vi "dfd_Get Filter Factor And Type From LM.vi"(8 "M":i32, 11 "L":i32) -> (0 "Factor":string, 3 "Type":string)   [LabVIEW 2017, in "NI_DigFilterLicensed.lvlib"]
uses:
  <vilib>/addons/Digital Filter Design/NI_DigFilterLicensed.lvlib
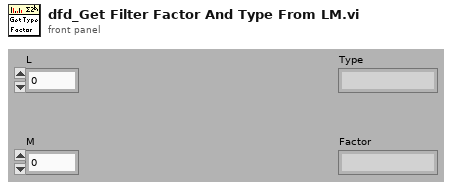
[diagram p1: front panel]
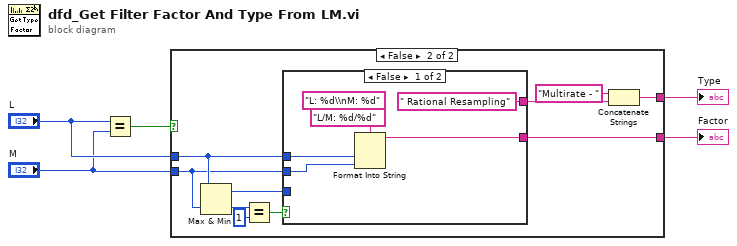
[diagram p0: block diagram]
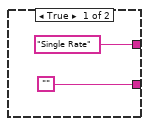
[diagram p2: hidden frame]
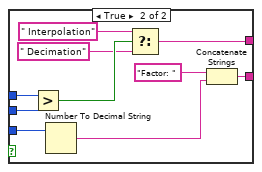
[diagram p3: hidden frame]
diagram:
  n1 = Equal?(x="L", y="M") -> (x = y?=w5:bool)
  n2 = case shown="False" w5 {
    tunnel: "L" -> [_ w13]
    tunnel: "M" -> [_ w12]
    tunnel: ["" w8] -> w1
    tunnel: ["Single Rate" w9] -> w2
    frame True {
    }
    frame False {
      n3 = Max & Min(x=w13, y=w12) -> (max(x,y)=w14:i32, min(x,y)=w16:i32)
      n4 = Equal?(x=w16, y=1) -> (x = y?=w17:bool)
      n5 = case shown="False" w17 {
        tunnel: w14 -> [_ w32]
        tunnel: [w20 w30] -> w8
        tunnel: w13 -> [w22 w28]
        tunnel: w12 -> [w21 w29]
        tunnel: [" Rational Resampling" w23] -> w11
        frame False {
          (unwired) "L: %d\\nM: %d" ("format string")
          n6 = Format Into String(format string="L/M: %d/%d", w22, w21) -> (resulting string=w20:string)  [unwired: 2 in, 1 out]
        }
        frame True {
          n7 = Greater?(x=w28, y=w29) -> (0:w26:bool)
          n8 = Number To Decimal String(number=w32) -> (decimal integer string=w31:string)  [unwired: 1 out]
          n9 = Select(t=" Interpolation", s=w26, f=" Decimation") -> (s? t:f=w23:string)
          n10 = Concatenate Strings("Factor: " ("string"), w31) -> (w30:string)
        }
      }
      n11 = Concatenate Strings("Multirate - " ("string"), w11) -> (w9:string)
    }
  }
  "Type" <- w2
  "Factor" <- w1
